vi "Get Profile Buffer(for Advanced Mode).vi"(3 "Data Size (0: Auto Size)":u32, 5 "Batch On-Off":bool) -> (0 "DWORD Buffer Size":u32, 2 "Profile Buffer":u32[](array[numeric]))   [LabVIEW 8.6, in "Keyence LJ-V7000.lvlib"]
uses:
  Keyence LJ-V7000.lvlib
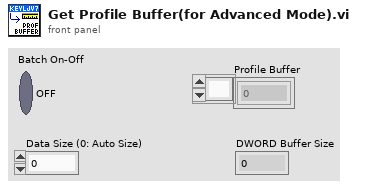
[diagram p1: front panel]
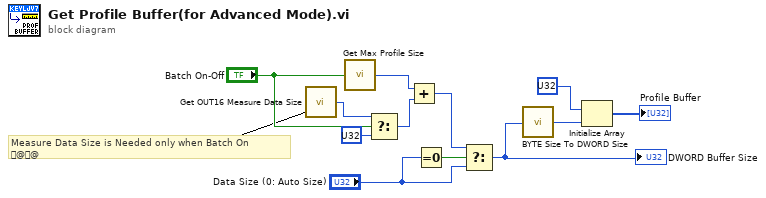
[diagram p0: block diagram]
diagram:
  # "Measure Data Size is Needed only when Batch On\n@@"
  n1 = call "Get OUT16 Measure Data Size.vi"() -> ("OUT16 Measure Data Size"=w5:u32)  [unwired: 1 in]
  n2 = call "Get Max Profile Size.vi"("Batch On-Off"="Batch On-Off") -> ("Profile Size"=w6:u32)  [unwired: 4 in]
  n3 = Select(t=w5, s="Batch On-Off", f=u32 ?) -> (s? t:f=w2:u32)
  n4 = Add(x=w6, y=w2) -> (x+y=w1:u32)
  n5 = Equal To 0?(x="Data Size (0: Auto Size)") -> (x = 0?=w9:bool)
  n6 = Select(t=w1, s=w9, f="Data Size (0: Auto Size)") -> (s? t:f=w8:u32)
  "DWORD Buffer Size" <- w8
  n7 = call "BYTE Size To DWORD Size.vi"("BYTE Size"=w8) -> ("DWORD Size"=w7:u32)
  n8 = Initialize Array(u32 ?, w7) -> (→"Profile Buffer":u32[])
